vi "Auto_Routine_BLUELeftTwoPieceTRAJ.vi"   [LabVIEW 2023]
uses:
  Arm2/ArmGetSetpointEnum.ctl
  Trajectory/TrajectoryGlobals.vi
  <vilib>/Rock Robotics/WPI/ThirdParty/JAS_Junk/TrajLib/Trajectory_Library.lvlib
types:
  T1 = typedef "ArmGetSetpointEnum.ctl" = enum16{"ArmFloorPickup", "ArmAmpDeposit", "ArmSpeakerShoot", "ArmStartPosition", "ArmRestPosition", "ArmSourceIntake", "ArmAwayShoot"}
  T2 = typedef "Trajectory_Library.lvlib/TRAJECTORY.ctl" = cluster{"TotalTImeSecs":dbl, "States":T3[]}
  T3 = typedef "Trajectory_Library.lvlib/TRAJ_STATE.ctl" = cluster{"TimeSeconds":dbl, "Velocity":dbl, "Acceleration":dbl, "POSE":T4, "Curvature":dbl}
  T4 = typedef "Trajectory_Library.lvlib/POSE2D.ctl" = cluster{"TRANSLATION":T5, "ROTATION":T6}
  T5 = typedef "Trajectory_Library.lvlib/TRANSLATION2D.ctl" = cluster{"X":dbl, "Y":dbl}
  T6 = typedef "Trajectory_Library.lvlib/ROTATION2D.ctl" = cluster{"VALUE":dbl, "COS":dbl, "SIN":dbl}
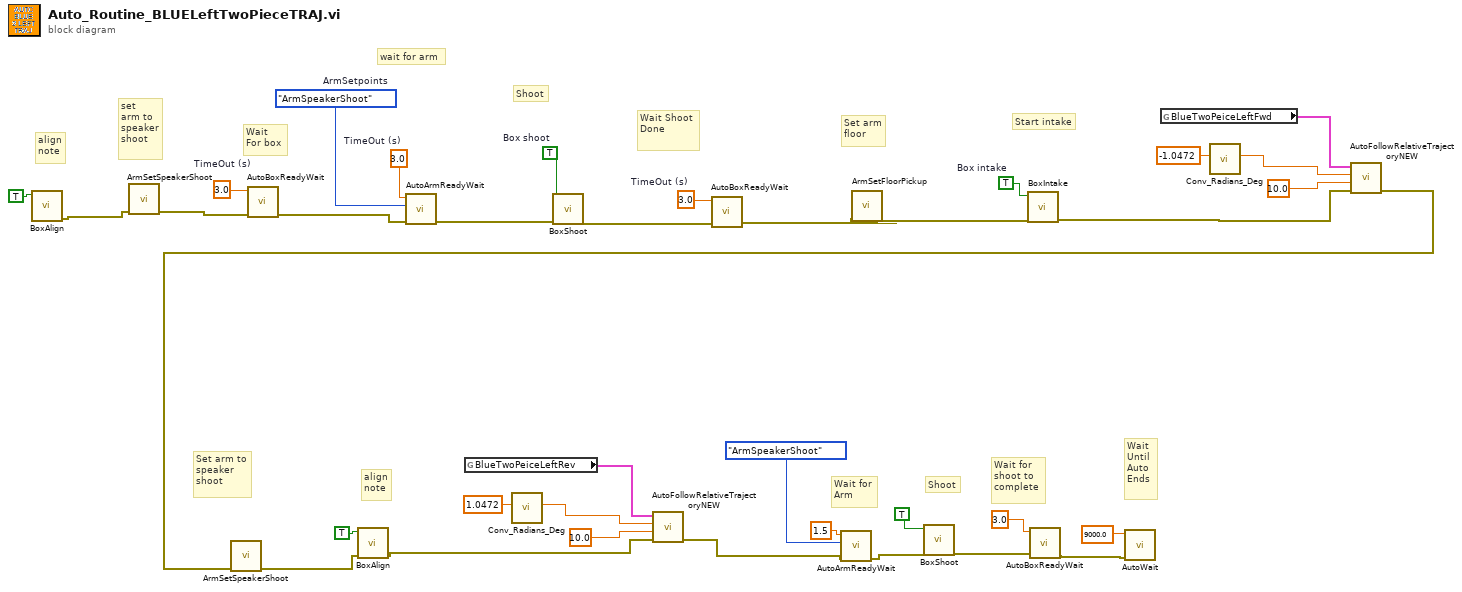
[diagram p0: block diagram]
diagram:
  w26 = 3.0  # TimeOut (s)
  w36 = TRUE  # Box intake
  w35 = TRUE  # Box shoot
  w34 = ArmGetSetpointEnum."ArmSpeakerShoot"  # ArmSetpoints
  w33 = 3.0  # TimeOut (s)
  w29 = 3.0  # TimeOut (s)
  # "align\nnote"
  # "Wait\nUntil\nAuto \nEnds"
  # "Wait for\nshoot to\ncomplete"
  # "Shoot"
  # "Wait for\nArm"
  # "Set arm to\nspeaker \nshoot"
  # "Start intake"
  # "Set arm\nfloor"
  # "Wait Shoot\nDone"
  # "Shoot"
  # "Wait\nFor box"
  # "set \narm to\nspeaker\nshoot"
  # "align\nnote"
  # "wait for arm"
  n1 = call "BoxAlign.vi"("box align"=TRUE) -> ("error out"=w27:errorcluster)  [unwired: 10 in]
  n2 = call "ArmSetSpeakerShoot.vi"("error in (no error)"=w27) -> ("error out"=w25:errorcluster)  [unwired: 10 in]
  n3 = call "AutoBoxReadyWait.vi"("error in (no error)"=w25, "TimeOut (s)"=w26) -> ("error out"=w24:errorcluster)  [unwired: 9 in]
  n4 = call "AutoArmReadyWait.vi"("error in (no error)"=w24, "ArmSetpoints"=w34, "TimeOut (s)"=w33) -> ("error out"=w30:errorcluster)  [unwired: 8 in]
  n5 = global read "TrajectoryGlobals.vi" "BlueTwoPeiceLeftRev"() -> (w9:T2)
  n6 = call <vilib>:"Conv_Radians_Deg.vi"("Radians"=1.0472) -> ("Degrees"=w7:dbl)  [unwired: 10 in]
  n7 = call "BoxShoot.vi"("error in (no error)"=w30, "Box shoot"=w35) -> ("error out"=w31:errorcluster)  [unwired: 9 in]
  n8 = call "AutoBoxReadyWait.vi"("error in (no error)"=w31, "TimeOut (s)"=w29) -> ("error out"=w23:errorcluster)  [unwired: 9 in]
  n9 = call "ArmSetFloorPickup.vi"("error in (no error)"=w23) -> ("error out"=w32:errorcluster)  [unwired: 10 in]
  n10 = call "BoxIntake.vi"("error in (no error)"=w32, "Box intake"=w36) -> ("error out"=w22:errorcluster)  [unwired: 9 in]
  n11 = global read "TrajectoryGlobals.vi" "BlueTwoPeiceLeftFwd"() -> (w21:T2)
  n12 = call <vilib>:"Conv_Radians_Deg.vi"("Radians"=-1.0472) -> ("Degrees"=w19:dbl)  [unwired: 10 in]
  n13 = call "AutoFollowRelativeTrajectoryNEW.vi"("error in (no error)"=w22, "TimeOut (s)"=10.0, "End Orientation"=w19, "Trajectory"=w21) -> ("error out"=w17:errorcluster)  [unwired: 7 in]
  n14 = call "ArmSetSpeakerShoot.vi"("error in (no error)"=w17) -> ("error out"=w2:errorcluster)  [unwired: 10 in]
  n15 = call "BoxAlign.vi"("error in (no error)"=w2, "box align"=TRUE) -> ("error out"=w1:errorcluster)  [unwired: 9 in]
  n16 = call "AutoFollowRelativeTrajectoryNEW.vi"("error in (no error)"=w1, "TimeOut (s)"=10.0, "End Orientation"=w7, "Trajectory"=w9) -> ("error out"=w5:errorcluster)  [unwired: 7 in]
  n17 = call "AutoArmReadyWait.vi"("error in (no error)"=w5, "ArmSetpoints"=ArmGetSetpointEnum."ArmSpeakerShoot", "TimeOut (s)"=1.5) -> ("error out"=w12:errorcluster)  [unwired: 8 in]
  n18 = call "BoxShoot.vi"("error in (no error)"=w12, "Box shoot"=TRUE) -> ("error out"=w15:errorcluster)  [unwired: 9 in]
  n19 = call "AutoBoxReadyWait.vi"("error in (no error)"=w15, "TimeOut (s)"=3.0) -> ("error out"=w4:errorcluster)  [unwired: 9 in]
  n20 = call "AutoWait.vi"("error in (no error)"=w4, "TimeOut (s)"=9000.0) -> ()  [unwired: 9 in, 1 out]
